vi "Galvo Test Harness.vi"() -> ()   [LabVIEW 2012]
uses:
  galvo_states.ctl
panel:
  in  "Cancel Button":bool
  in  "Refresh Button":bool
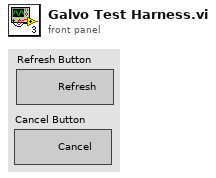
[diagram p1: front panel]
types:
  T1 = typedef "galvo_states.ctl" = enum16{"Reset", "Reset Galvos?", "Center Galvos", "Register Callback", "Get Scan Parameters", "Show", "Initialize", "Run Raster", "Load Raster", "Run Circle", "Shutdown"}
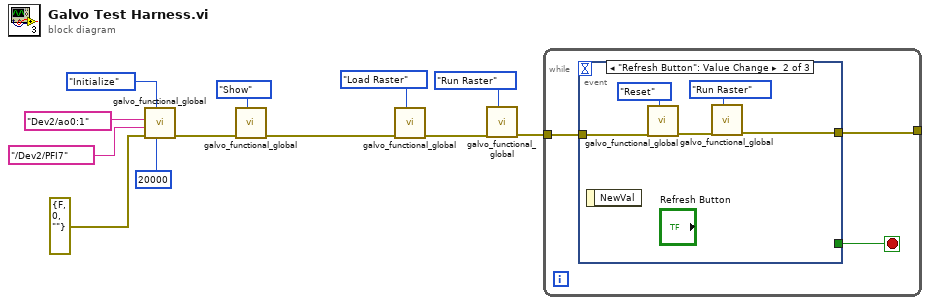
[diagram p0: block diagram]
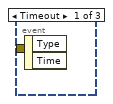
[diagram p2: hidden frame]
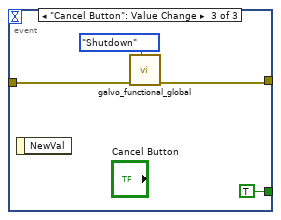
[diagram p3: hidden frame]
diagram:
  n1 = call "galvo_functional_global.vi"("Est Sweep Speed"=20000, "State"=galvo_states."Initialize", "error in (no error)"=errorcluster {"status"=FALSE, "code"=0, "source"=""} ("error constant"), "Trigger Source"=tag "/Dev2/PFI7", "Analog Output"=tag "Dev2/ao0:1" ("Channels")) -> ("error out"=w4:errorcluster)  [unwired: 5 in, 1 out]
  n2 = call "galvo_functional_global.vi"("State"=galvo_states."Show", "error in (no error)"=w4) -> ("error out"=w3:errorcluster)  [unwired: 8 in, 1 out]
  n3 = call "galvo_functional_global.vi"("State"=galvo_states."Load Raster", "error in (no error)"=w3) -> ("error out"=w8:errorcluster)  [unwired: 8 in, 1 out]
  n4 = call "galvo_functional_global.vi"("State"=galvo_states."Run Raster", "error in (no error)"=w8) -> ("error out"=w6:errorcluster)  [unwired: 8 in, 1 out]
  n5 = while {
    tunnel: w6 -> [w15]
    tunnel: [w14] -> _
    stop <- w13 stop-if-true
    n6 = event shown="[1] \"Refresh Button\": Value Change" {
      selector: _ -> [_ _ _]
      dyn-events: _ -> [_ _ _]
      timeout: _ -> [_ _ _]
      tunnel: w15 -> [_ w20 w23]
      tunnel: [_ w16 w22] -> w14
      tunnel: [_ _ TRUE] -> w13
      event Timeout {
        n7 = event-data() -> ()  [unwired: 1 in, 2 out]
      }
      event "Refresh Button": Value Change {
        n8 = event-data() -> ()  [unwired: 1 in, 1 out]
        n9 = call "galvo_functional_global.vi"("State"=galvo_states."Reset", "error in (no error)"=w20) -> ("error out"=w18:errorcluster)  [unwired: 8 in, 1 out]
        n10 = call "galvo_functional_global.vi"("State"=galvo_states."Run Raster", "error in (no error)"=w18) -> ("error out"=w16:errorcluster)  [unwired: 8 in, 1 out]
      }
      event "Cancel Button": Value Change {
        n11 = event-data() -> ()  [unwired: 1 in, 1 out]
        n12 = call "galvo_functional_global.vi"("State"=galvo_states."Shutdown", "error in (no error)"=w23) -> ("error out"=w22:errorcluster)  [unwired: 8 in, 1 out]
      }
    }
  }
